vi "Task_robot_position_Reference.vi"(8 "error in (no error)":errorcluster caption="错误输入（无错误）", 10 "值(信号)":T1, 11 "Map输入":refnum<class "Map.lvclass">) -> (0 "error out":errorcluster caption="错误输出", 3 "Map输出":refnum<class "Map.lvclass">)   [LabVIEW 2014, in "Map.lvlib" / "Map.lvclass"]
uses:
  Map.lvclass
  MapBuilder/Robot_Position.ctl
  Map.lvclass/Map.ctl
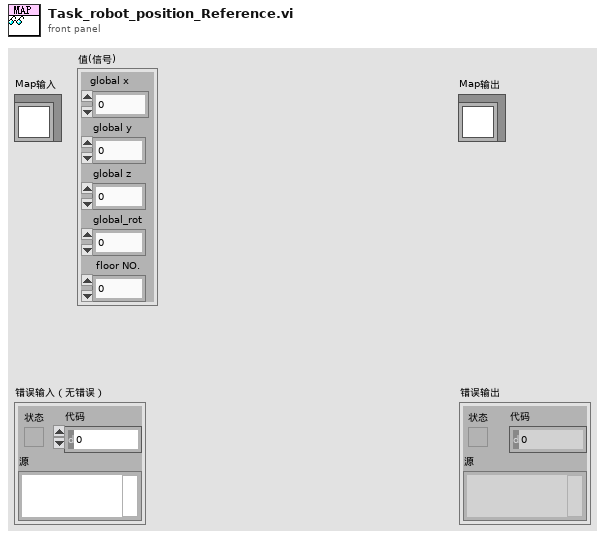
[diagram p1: front panel]
types:
  T1 = typedef "Robot_Position.ctl" = cluster{"global x":dbl, "global y":dbl, "global z":dbl, "global_rot":dbl, " floor NO.":dbl}
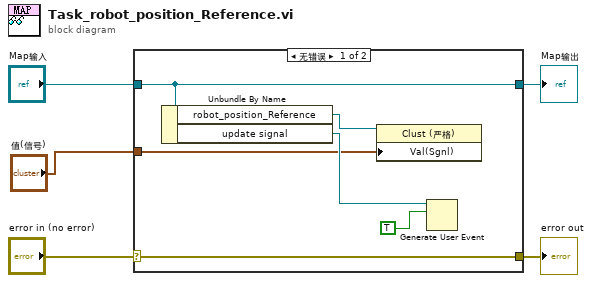
[diagram p0: block diagram]
diagram:
  n1 = case shown="无错误" "error in (no error)" {
    selector: "error in (no error)" -> [w11 w12]
    tunnel: [w11 w12] -> w4
    tunnel: [w10 w13] -> w2
    tunnel: "Map输入" -> [w10 w13]
    tunnel: "值(信号)" -> [w6 _]
    frame No Error {
      n2 = Unbundle By Name(w10) -> ("robot_position_Reference"=w9:refnum<vi>, "update signal"=w7:refnum<user-event>)
      n3 = property class="Clust (严格)"(reference=w9, "Val(Sgnl)"=w6) -> ()  [unwired: 1 in, 2 out]
      n4 = Generate User Event(user event=w7, event data cluster=TRUE ("事件数据")) -> ()  [unwired: 2 in, 2 out]
    }
    frame Error {
    }
  }
  "error out" <- w4
  "Map输出" <- w2
